vi "Get - LMS Filter Coefs and Signals.vi"(0 "reference in":refnum<class "AdvSigProc.lvclass">, 5 "error in (no error)":errorcluster) -> (11 "Filter Coefs":dbl[](array[numeric]), 13 "LMS Filtered Signals":waveform(dbl)[](array[waveform]), 14 "reference out":refnum<class "AdvSigProc.lvclass">, 19 "error out":errorcluster)   [LabVIEW 2020, in "AdvSigProc.lvclass"]
uses:
  AdvSigProc.lvclass
  API/GSwFormDSP_class/GSwFormDSP.lvclass
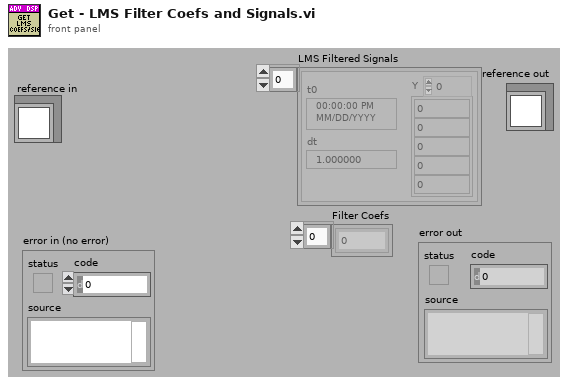
[diagram p1: front panel]
types:
  T1 = typedef "AdvSigProc.lvclass/ObjectAttributes.ctl" = cluster{"Time Data":cluster{"New Time Data Obj?":bool, "GSwFormDSP":refnum<class "GSwFormDSP.lvclass">}, "LMS Parameters":T2}
  T2 = typedef "AdvSigProc.lvclass/LMS.ctl" = cluster{"adaptive filter Ref":refnum<k20>, "Filtered Signals":refnum<class "GSwFormDSP.lvclass">, "Filter Coefs":dbl[], "Input Parameters":T3, "Iteration Metrics":T4[]}
  T3 = typedef "AdvSigProc.lvclass/LMS Input Parameters.ctl" = cluster{"Type":enum16{"Normalized LMS", "LMS", "FIR Sign LMS", "FIR Fast Block LMS", "RLS", "QR - RLS"}, "Filter Class":enum16{"Noise Cancelling (BGN Ref)", "Noise Cancelling (Speech Ref)"}, "Filter Length":i32, "µ Parameters":cluster{"Type":enum16{"User Input", "Auto µ"}, "step size":dbl}, "Iterations":cluster{"Current":i32, "Maximum":i32}}
  T4 = typedef "AdvSigProc.lvclass/Iteration Metrics.ctl" = cluster{"Name":string, "Max":dbl, "Min":dbl, "Values History":dbl[]}
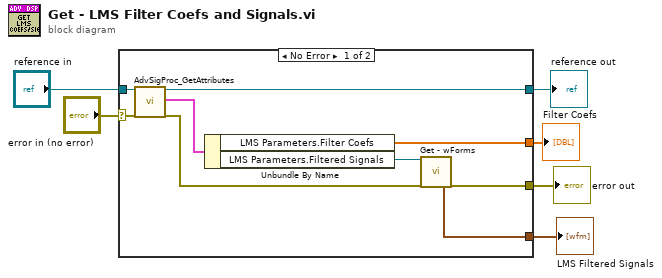
[diagram p0: block diagram]
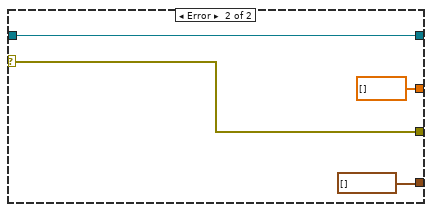
[diagram p2: hidden frame]
diagram:
  n1 = case shown="No Error" "error in (no error)" {
    selector: "error in (no error)" -> [w15 w19]
    tunnel: [w9 w19] -> w5
    tunnel: [w14 w18] -> w3
    tunnel: "reference in" -> [w12 w18]
    tunnel: [w8 dbl[] [] ("Filter Coefs")] -> w1
    tunnel: [w7 waveform(dbl)[] [] ("wForms")] -> w2
    frame No Error {
      n2 = call "AdvSigProc_GetAttributes.vi"("reference in"=w12, "error in (no error)"=w15) -> ("reference out"=w14:refnum<class "AdvSigProc.lvclass">, "attributes"=w13:T1, "error out"=w10:errorcluster)  [unwired: 14 in, 1 out]
      n3 = Unbundle By Name(w13) -> ("LMS Parameters.Filter Coefs"=w8:dbl[], "LMS Parameters.Filtered Signals"=w11:refnum<class "GSwFormDSP.lvclass">)
      n4 = call-dynamic "Get - wForms.vi"("reference in"=w11, "error in (no error)"=w10) -> ("wForms"=w7:waveform(dbl)[], "error out"=w9:errorcluster)  [unwired: 14 in, 2 out]
    }
    frame Error {
    }
  }
  "error out" <- w5
  "reference out" <- w3
  "LMS Filtered Signals" <- w2
  "Filter Coefs" <- w1
